vi "lens.vi"(7 "y_shift":dbl, 9 "x_shift":dbl, 10 "focal_length":dbl=0.5, 11 "field":T1) -> (3 "field out":T1)   [LabVIEW 2012, in "LightPipes.lvlib"]
doc: "__declspec(dllexport) void lens(FIELD* field, double focal_length, double x_shift, double y_shift);"
uses:
  LightPipes.lvlib
  Lightpipes.dll
panel:
  out "error out":errorcluster
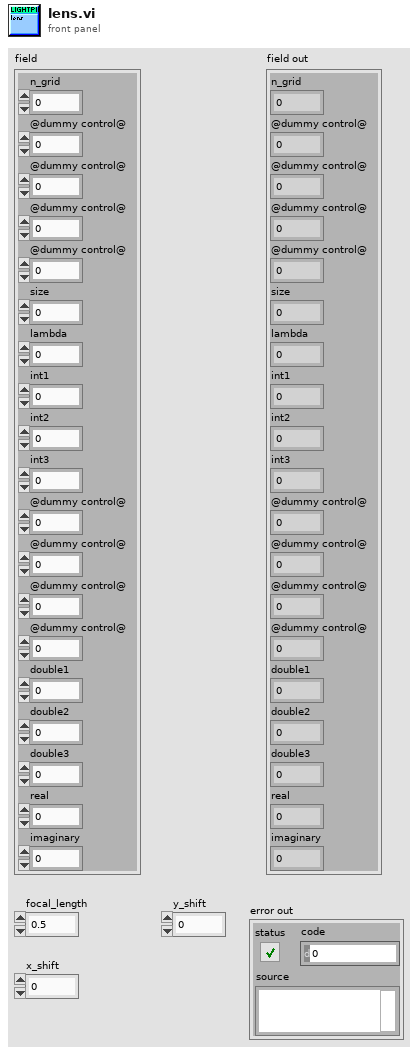
[diagram p1: front panel]
types:
  T1 = cluster{"n_grid":i32, "@dummy control@":i8, "@dummy control@":i8, "@dummy control@":i8, "@dummy control@":i8, "size":dbl, "lambda":dbl, "int1":i32, "int2":i32, "int3":i32, "@dummy control@":i8, "@dummy control@":i8, "@dummy control@":i8, "@dummy control@":i8, "double1":dbl, "double2":dbl, "double3":dbl, "real":u32, "imaginary":u32}
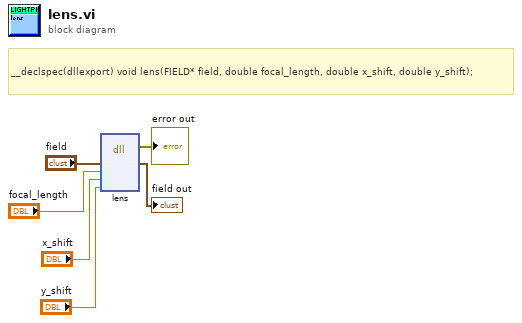
[diagram p0: block diagram]
diagram:
  # "__declspec(dllexport) void lens(FIELD* field, double focal_length, double x_shift, double y_shift);"
  n1 = dll-call lib="C:/Users/Tri/Documents/Gerchberg/LightPipes.*" fn="lens"("field"="field", "focal_length"="focal_length", "x_shift"="x_shift", "y_shift"="y_shift") -> (error out=→"error out":errorcluster, "field"=→"field out":T1)  [unwired: 7 in, 1 out]
